vi "Part 1.vi"(11 "Input":string) -> (3 "Output":i64)   [LabVIEW 2021]
uses:
  <userlib>/_OpenG.lib/md5/md5.llb/MD5 Message Digest (Hexadecimal String)__ogtk.vi
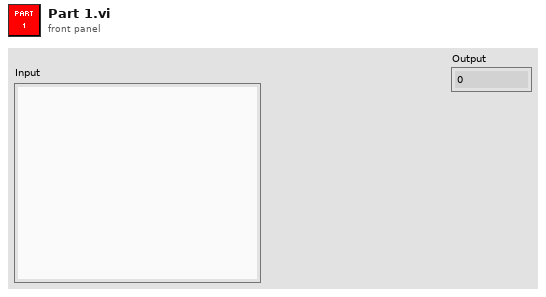
[diagram p1: front panel]
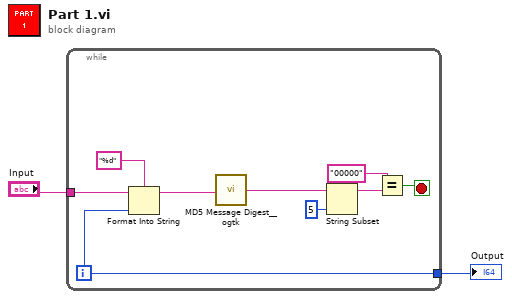
[diagram p0: block diagram]
diagram:
  n1 = while {
    tunnel: "Input" -> [w11]
    tunnel: [w3] -> w1
    i -> [w3]
    stop <- w4 stop-if-true
    n2 = Format Into String(format string="%d", initial string=w11, w3) -> (resulting string=w9:string)  [unwired: 1 in, 1 out]
    n3 = call-poly <userlib>:"MD5 Message Digest__ogtk.vi"("Message"=w9) -> ("MD5 Message Digest"=w8:string)
    n4 = String Subset(string=w8, length (rest)=5 ("length (rest)")) -> (substring=w6:string)  [unwired: 1 in]
    n5 = Equal?(x="00000", y=w6) -> (x = y?=w4:bool)
  }
  "Output" <- w1
